vi "MFC_Set.vi"(8 "error in":errorcluster, 9 "Setpoint":dbl format="%_4g", 10 "Previous Setpoint":dbl=nan format="%_4g", 11 "Communication Settings":T2={"Unit ID"="A", "Baud Rate"=enum."19200", "VISA Sesssion In"="ASRL1::INSTR"}) -> (0 "error out":errorcluster, 1 "Delay":dbl, 2 "Data Cluster":T1)   [LabVIEW 2019]
panel:
  out "Controller Info out":T3={"Controller Full Scale"=nan, "Controller Select"=0, "Control Range"=enum."Normal"} {"Controller Select" items=["No controller"=0, "Volumetric Flow"=36, "Mass Flow"=37, "Absolute Pressure"=34, "Gauge Pressure"=38, "Differential Pressure"=39]}
  out "Data Frame Format":T4
  # "Totalizer Timer"
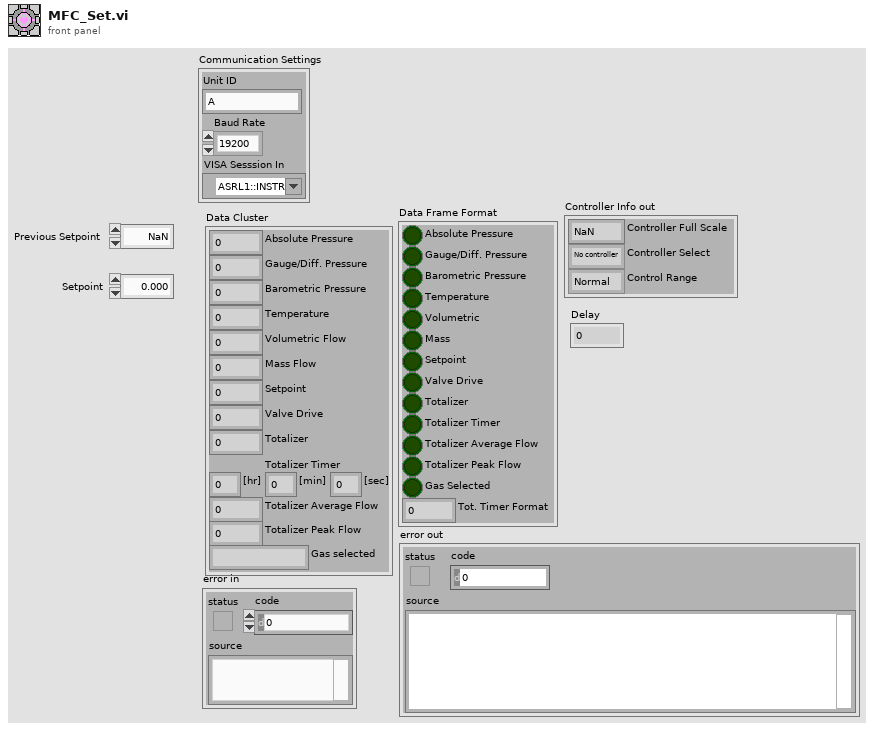
[diagram p1: front panel]
types:
  T1 = cluster{"Absolute Pressure":dbl, "Gauge/Diff. Pressure":dbl, "Barometric Pressure":dbl, "Temperature":dbl, "Volumetric Flow":dbl, "Mass Flow":dbl, "Setpoint":dbl, "Valve Drive":dbl, "Totalizer":dbl, "[hr]":dbl, "[min]":dbl, "[sec]":dbl, "Totalizer Average Flow":dbl, "Totalizer Peak Flow":dbl, "Gas selected":string}
  T2 = cluster{"Unit ID":string, "Baud Rate":enum8{"2400", "9600", "19200", "38400", "57600", "115200", "Unknown"}, "VISA Sesssion In":refnum<visa-resource-name>}
  T3 = cluster{"Controller Full Scale":dbl, "Controller Select":u16, "Control Range":enum16{"Normal", "Inverted", "Bidirectional", "Unknown"}}
  T4 = cluster{"Absolute Pressure":bool, "Gauge/Diff. Pressure":bool, "Barometric Pressure":bool, "Temperature":bool, "Volumetric":bool, "Mass":bool, "Setpoint":bool, "Valve Drive":bool, "Totalizer":bool, "Totalizer Timer":bool, "Totalizer Average Flow":bool, "Totalizer Peak Flow":bool, "Gas Selected":bool, "Tot. Timer Format":u16}
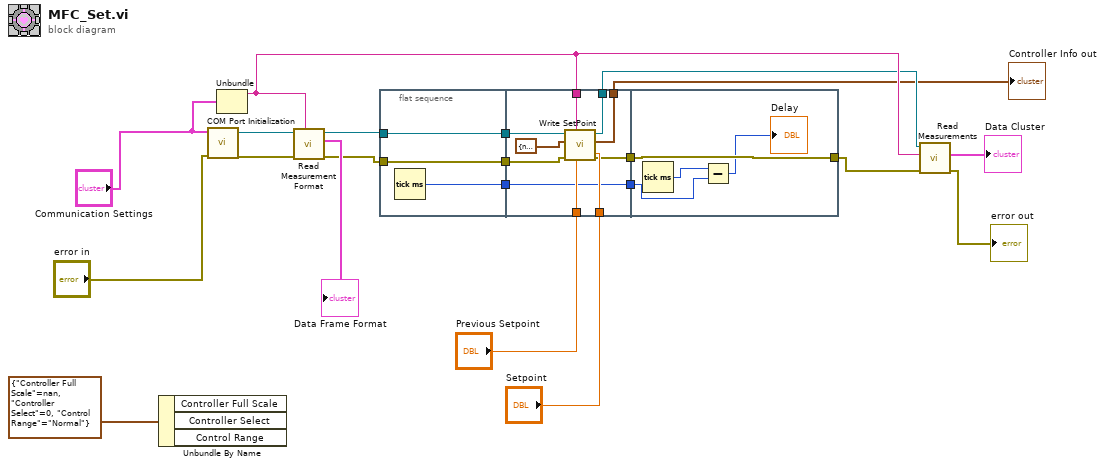
[diagram p0: block diagram]
diagram:
  n1 = Unbundle By Name(T3 {"Controller Full Scale"=nan, "Controller Select"=0, "Control Range"=enum."Normal"} ("Controller Info out")) -> ()  [unwired: 3 out]
  n2 = call <instrlib>:"COM Port Initialization.vi"("error in (no error)"="error in", "Communication Settings"="Communication Settings") -> ("error out"=w15:errorcluster, "VISA Session Out"=w16:refnum<visa-resource-name>)  [unwired: 8 in]
  n3 = Unbundle("Communication Settings") -> ("Unit ID"=w3:string)  [unwired: 2 out]
  n4 = call <instrlib>:"Read Measurement Format.vi"("Unit ID (A)"=w3, "error in"=w15, "VISA Session In"=w16) -> ("error out"=w7:errorcluster, "Data Frame Format"=→"Data Frame Format":T4, "VISA Session Out"=w6:refnum<visa-resource-name>)  [unwired: 6 in]
  n5 = flat-sequence {
    tunnel: w7 -> [w23]
    tunnel: w6 -> [w24]
    tunnel: [w24] -> w21
    tunnel: [w23] -> w20
    tunnel: [w22] -> w19
    tunnel: "Previous Setpoint" -> [w33]
    tunnel: "Setpoint" -> [w32]
    tunnel: [w31] -> w18
    tunnel: w21 -> [w34]
    tunnel: w20 -> [w30]
    tunnel: [w29] -> w17
    tunnel: w19 -> [w29]
    tunnel: w3 -> [w27]
    tunnel: [w26] -> w2
    tunnel: [w25] -> w1
    tunnel: [w38] -> w5
    tunnel: w18 -> [w38]
    tunnel: w17 -> [w36]
    frame #0 {
      n6 = Tick Count (ms)() -> (millisecond timer value=w22:u32)
    }
    frame #1 {
      n7 = call <instrlib>:"Write SetPoint.vi"("Setpoint"=w32, "Previous Setpoint"=w33, "Unit ID (A)"=w27, "error in"=w30, "Controller Info out"=T3 {"Controller Full Scale"=nan, "Controller Select"=0, "Control Range"=enum."Normal"}, "VISA Session In"=w34) -> ("error out"=w31:errorcluster, "Controller Info out"=w25:T3, "VISA Session Out"=w26:refnum<visa-resource-name>)  [unwired: 2 in, 1 out]
    }
    frame #2 {
      n8 = Tick Count (ms)() -> (millisecond timer value=w37:u32)
      n9 = Subtract(x=w37, y=w36) -> (x-y=→"Delay":u32)
    }
  }
  n10 = call <instrlib>:"Read Measurements.vi"("error in"=w5, "Unit ID (A)"=w3, "VISA Session In"=w2) -> ("error out"=→"error out":errorcluster, "Data Cluster"=→"Data Cluster":T1)  [unwired: 1 in, 6 out]
  "Controller Info out" <- w1
